vi "Auto_filename.vi"(1 "Filename Max length":i32=28, 2 "Prefix":string) -> (0 "Filename":string)   [LabVIEW 2020]
uses:
  Results_plotter_Global.vi
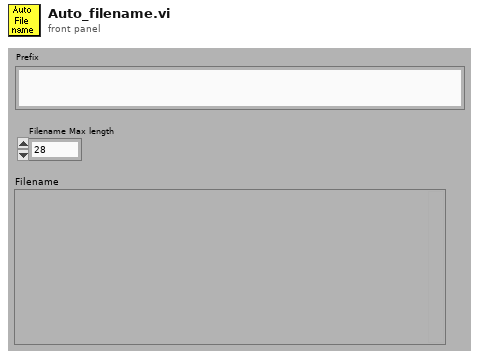
[diagram p1: front panel]
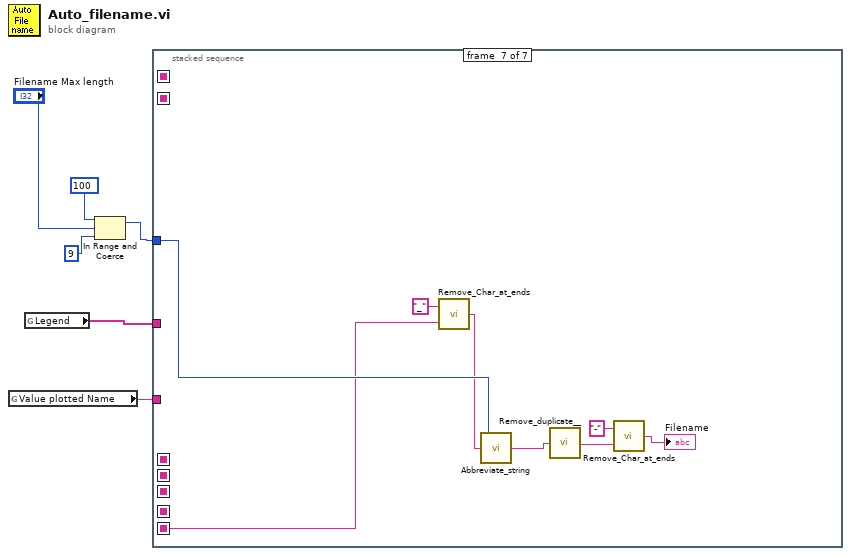
[diagram p0: block diagram]
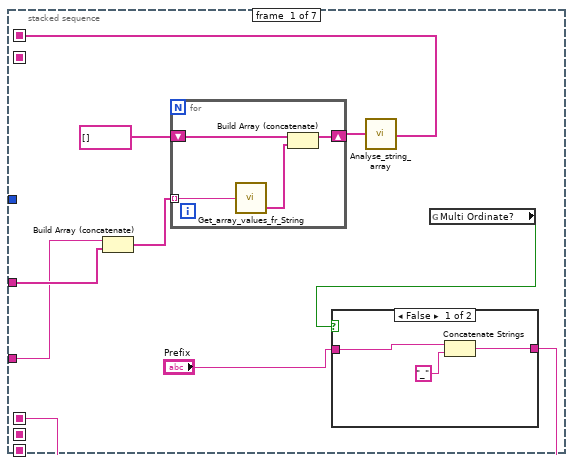
[diagram p2: hidden frame]
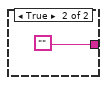
[diagram p3: hidden frame]
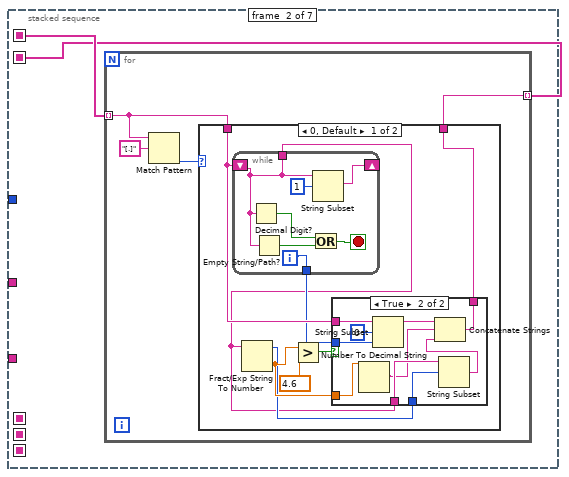
[diagram p4: hidden frame]
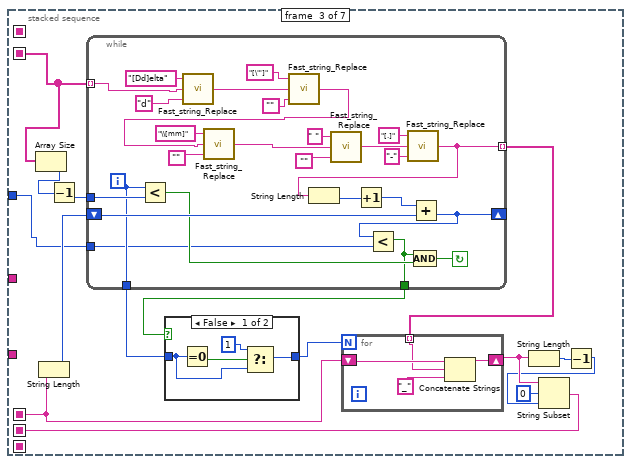
[diagram p7: hidden frame]
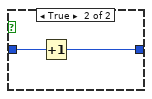
[diagram p8: hidden frame]
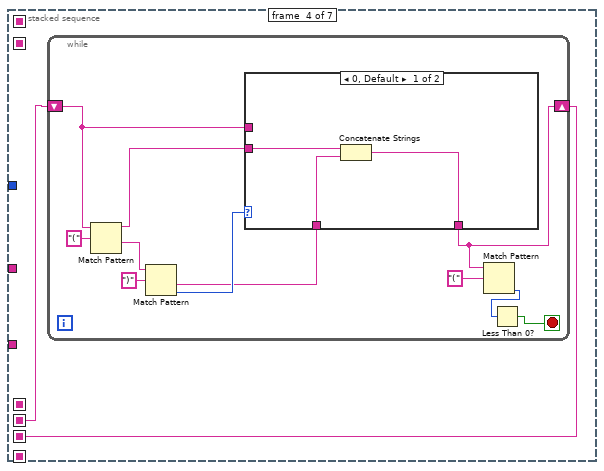
[diagram p9: hidden frame]
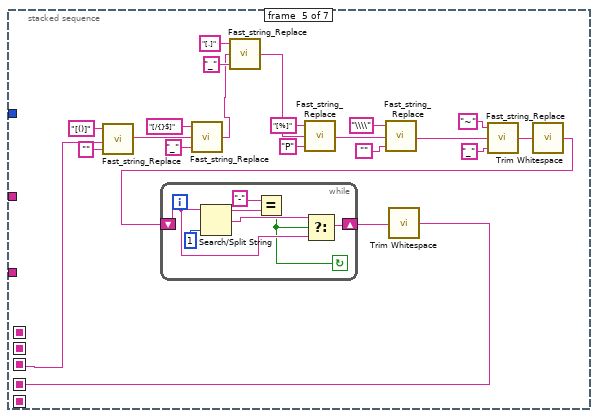
[diagram p11: hidden frame]
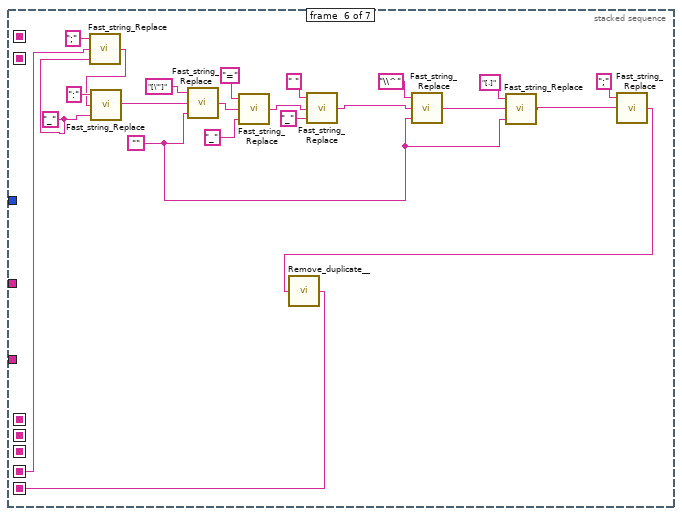
[diagram p12: hidden frame]
diagram:
  n1 = global read "Results_plotter_Global.vi" "Value plotted Name"() -> (w5:string)
  n2 = global read "Results_plotter_Global.vi" "Legend"() -> (w6:string[])
  n3 = In Range and Coerce(upper limit=100 ("length (rest)"), x="Filename Max length", lower limit=9) -> (coerced(x)=w1:i32)  [unwired: 1 out]
  n4 = stacked-sequence {
    seq-local: [_ w24 _ _ _ _ _] -> [_ _ w70 _ _ _ _]
    seq-local: [w13 _ _ _ _ _ _] -> [_ w25 _ _ _ _ _]
    seq-local: [w11 _ _ _ _ _ _] -> [_ _ w63 _ _ _ _]
    seq-local: [_ _ _ w108 _ _ _] -> [_ _ _ _ w139 _ _]
    seq-local: [_ _ _ _ w145 _ _] -> [_ _ _ _ _ w161 _]
    seq-local: [_ _ w57 _ _ _ _] -> [_ _ _ w109 _ _ _]
    seq-local: [_ _ _ _ _ w166 _] -> [_ _ _ _ _ _ w176]
    tunnel: w6 -> [w9 _ _ _ _ _ _]
    tunnel: w5 -> [w8 _ _ _ _ _ _]
    tunnel: w1 -> [_ _ w58 _ _ _ w183]
    frame #0 {
      n5 = Build Array (concatenate)(w8, w9) -> (w7:string[])
      n6 = for {
        tunnel: w7 -> [w23] mode=indexing
        shift-right: [w21] -> w14
        shift-left: string[] [] ("String array") -> [w22]
        n7 = call "Get_array_values_fr_String.vi"("String Value"=w23) -> ("String array"=w20:string[])  [unwired: 1 out]
        n8 = Build Array (concatenate)(w22, w20) -> (w21:string[])
      }
      n9 = call "Analyse_string_array.vi"("String array"=w14) -> ("Unique strings"=w13:string[])  [unwired: 2 out]
      n10 = global read "Results_plotter_Global.vi" "Multi Ordinate?"() -> (w12:bool)
      n11 = case shown="False" w12 {
        tunnel: [w17 ""] -> w11
        tunnel: "Prefix" -> [w16 _]
        frame False {
          n12 = Concatenate Strings(w16, "_" ("string")) -> (w17:string)
        }
        frame True {
        }
      }
    }
    frame #1 {
      n13 = for {
        tunnel: w25 -> [w27] mode=indexing
        tunnel: [w26] -> w24 mode=indexing
        n14 = Match Pattern(string=w27, regular expression="[.]") -> (offset past match=w28:i32)  [unwired: 4 out]
        n15 = case shown="0, Default" w28 {
          tunnel: [w31 w56] -> w26
          tunnel: w27 -> [w35 w56]
          frame 0, Default {
            n16 = while {
              shift-right: [w54] -> _
              shift-left: w35 -> [w49]
              tunnel: [w50] -> w34
              tunnel: [w49] -> w30
              i -> [w50]
              stop <- w53 stop-if-true
              n17 = Decimal Digit?(1:w49) -> (0:w52:bool)
              n18 = Empty String/Path?(string/path=w49) -> (empty?=w51:bool)
              n19 = Or(x=w52, y=w51) -> (x .or. y?=w53:bool)
              n20 = String Subset(string=w49, offset (0)=1) -> (substring=w54:string)  [unwired: 1 out]
            }
            n21 = Fract/Exp String To Number(string=w30) -> (offset past number=w32:i32, number=w33:dbl)  [unwired: 3 out]
            n22 = Greater?(x=w33, y=4.6) -> (0:w36:bool)
            n23 = case shown="True" w36 {
              tunnel: w35 -> [w38 w47]
              tunnel: w34 -> [_ w46]
              tunnel: w33 -> [_ w45]
              tunnel: w32 -> [_ w44]
              tunnel: w30 -> [_ w43]
              tunnel: [w38 w39] -> w31
              frame False {
              }
              frame True {
                n24 = Number To Decimal String(number=w45) -> (decimal integer string=w41:string)  [unwired: 1 out]
                n25 = String Subset(string=w47, offset (0)=0, length (rest)=w46) -> (substring=w42:string)
                n26 = String Subset(string=w43, offset (0)=w44) -> (substring=w40:string)  [unwired: 1 out]
                n27 = Concatenate Strings(w42, w41, w40) -> (w39:string)
              }
            }
          }
          frame -1 {
          }
        }
      }
    }
    frame #2 {
      n28 = Array Size(array=w70) -> (size(s)=w69:i32)
      n29 = String Length(string=w63) -> (length=w71:i32)
      n30 = Decrement(x=w69) -> (x-1=w68:i32)
      n31 = while {
        tunnel: w70 -> [w88] mode=indexing
        shift-right: [w96] -> _
        shift-left: w71 -> [w98]
        tunnel: w68 -> [w97]
        tunnel: [w92] -> w67
        tunnel: [w91] -> w66
        tunnel: [w90] -> w64 mode=indexing
        tunnel: w58 -> [w82]
        i -> [w91]
        stop <- w94 continue-if-true
        n32 = Less?(x=w91, y=w97) -> (x < y?=w93:bool)
        n33 = call "Fast_string_Replace.vi"("Replace match with:"="d", "Input String"=w88, "regular expression"="[Dd]elta") -> ("Output String"=w85:string)  [unwired: 2 out]
        n34 = call "Fast_string_Replace.vi"("Replace match with:"="", "Input String"=w85, "regular expression"="[\"']") -> ("Output String"=w83:string)  [unwired: 2 out]
        n35 = call "Fast_string_Replace.vi"("Replace match with:"="", "Input String"=w83, "regular expression"="\\[mm]") -> ("Output String"=w103:string)  [unwired: 2 out]
        n36 = call "Fast_string_Replace.vi"("Replace match with:"="", "Input String"=w103, "regular expression"=" ") -> ("Output String"=w101:string)  [unwired: 2 out]
        n37 = call "Fast_string_Replace.vi"("Replace match with:"="-", "Input String"=w101, "regular expression"="[.]") -> ("Output String"=w90:string)  [unwired: 2 out]
        n38 = String Length(string=w90) -> (length=w99:i32)
        n39 = Increment(x=w99) -> (x+1=w95:i32)
        n40 = Add(x=w95, y=w98) -> (x+y=w96:i32)
        n41 = Less?(x=w96, y=w82) -> (x < y?=w92:bool)
        n42 = Compound Arithmetic op=AND(w92, w93) -> (w94:bool)
      }
      n43 = case shown="False" w67 {
        tunnel: [w76 w80] -> w65
        tunnel: w66 -> [w78 w81]
        frame False {
          n44 = Equal To 0?(x=w78) -> (x = 0?=w79:bool)
          n45 = Select(t=1, s=w79, f=w78) -> (s? t:f=w76:i32)
        }
        frame True {
          n46 = Increment(x=w81) -> (x+1=w80:i32)
        }
      }
      n47 = for {
        N: w65 -> [_]
        shift-right: [w72] -> w61
        shift-left: w63 -> [w75]
        tunnel: w64 -> [w74] mode=indexing
        n48 = Concatenate Strings(w75, w74, "_" ("string")) -> (w72:string)
      }
      n49 = String Length(string=w61) -> (length=w62:i32)
      n50 = Decrement(x=w62) -> (x-1=w59:i32)
      n51 = String Subset(string=w61, offset (0)=0, length (rest)=w59) -> (substring=w57:string)
    }
    frame #3 {
      n52 = while {
        shift-right: [w112] -> w108
        shift-left: w109 -> [w114]
        stop <- w110 stop-if-true
        n53 = Match Pattern(string=w114, regular expression="(") -> (before substring=w116:string, after substring=w118:string)  [unwired: 3 out]
        n54 = Match Pattern(string=w118, regular expression=")") -> (after substring=w115:string, offset past match=w117:i32)  [unwired: 3 out]
        n55 = case shown="0, Default" w117 {
          tunnel: [w121 w124] -> w112
          tunnel: w114 -> [_ w124]
          tunnel: w116 -> [w123 _]
          tunnel: w115 -> [w122 _]
          frame 0, Default {
            n56 = Concatenate Strings(w123, w122) -> (w121:string)
          }
          frame -1 {
          }
        }
        n57 = Match Pattern(string=w112, regular expression="(") -> (offset past match=w111:i32)  [unwired: 4 out]
        n58 = Less Than 0?(x=w111) -> (x < 0?=w110:bool)
      }
    }
    frame #4 {
      n59 = call "Fast_string_Replace.vi"("Replace match with:"="", "Input String"=w139, "regular expression"="[()]") -> ("Output String"=w140:string)  [unwired: 2 out]
      n60 = call "Fast_string_Replace.vi"("Replace match with:"="_", "Input String"=w140, "regular expression"="[/{}$]") -> ("Output String"=w126:string)  [unwired: 2 out]
      n61 = call "Fast_string_Replace.vi"("Replace match with:"="_", "Input String"=w126, "regular expression"="[.]") -> ("Output String"=w125:string)  [unwired: 2 out]
      n62 = call "Fast_string_Replace.vi"("Replace match with:"="P", "Input String"=w125, "regular expression"="[%]") -> ("Output String"=w134:string)  [unwired: 2 out]
      n63 = call "Fast_string_Replace.vi"("Replace match with:"="", "Input String"=w134, "regular expression"="\\\\") -> ("Output String"=w130:string)  [unwired: 2 out]
      n64 = call "Fast_string_Replace.vi"("Replace match with:"="_", "Input String"=w130, "regular expression"="~") -> ("Output String"=w129:string)  [unwired: 2 out]
      n65 = call <vilib>:"Trim Whitespace.vi"("string"=w129) -> ("trimmed string"=w138:string)  [unwired: 1 in]
      n66 = while {
        shift-left: w138 -> [w149]
        shift-right: [w147] -> w146
        stop <- w148 continue-if-true
        n67 = Search/Split String(string=w149, offset (0)=1 ("length")) -> (substring before match=w152:string, match + rest of string=w150:string)  [unwired: 2 out]
        n68 = Equal?(x="-", y=w152) -> (x = y?=w148:bool)
        n69 = Select(t=w150, s=w148, f=w149) -> (s? t:f=w147:string)
      }
      n70 = call <vilib>:"Trim Whitespace.vi"("string"=w146) -> ("trimmed string"=w145:string)  [unwired: 1 in]
    }
    frame #5 {
      w162 = "_" ("Replace match with:")
      w157 = ""
      n71 = call "Fast_string_Replace.vi"("Replace match with:"=w162, "Input String"=w161, "regular expression"=";") -> ("Output String"=w160:string)  [unwired: 2 out]
      n72 = call "Fast_string_Replace.vi"("Replace match with:"=w162, "Input String"=w160, "regular expression"=":") -> ("Output String"=w171:string)  [unwired: 2 out]
      n73 = call "Fast_string_Replace.vi"("Replace match with:"=w157, "Input String"=w171, "regular expression"="[\"']") -> ("Output String"=w168:string)  [unwired: 2 out]
      n74 = call "Fast_string_Replace.vi"("Replace match with:"="_", "Input String"=w168, "regular expression"="=") -> ("Output String"=w167:string)  [unwired: 2 out]
      n75 = call "Fast_string_Replace.vi"("Replace match with:"="_", "Input String"=w167, "regular expression"=" ") -> ("Output String"=w164:string)  [unwired: 2 out]
      n76 = call "Fast_string_Replace.vi"("Replace match with:"=w157, "Input String"=w164, "regular expression"="\\^") -> ("Output String"=w158:string)  [unwired: 2 out]
      n77 = call "Fast_string_Replace.vi"("Replace match with:"=w157, "Input String"=w158, "regular expression"="[.]") -> ("Output String"=w155:string)  [unwired: 2 out]
      n78 = call "Fast_string_Replace.vi"("Input String"=w155, "regular expression"=";") -> ("Output String"=w154:string)  [unwired: 1 in, 2 out]
      n79 = call "Remove_duplicate__.vi"("Output String"=w154) -> ("String"=w166:string)
    }
    frame #6 {
      n80 = call "Remove_Char_at_ends.vi"("String in"=w176, "Characters to remove"="_" ("Character to remove")) -> ("String out"=w182:string)
      n81 = call "Abbreviate_string.vi"("Input String"=w182, "Max String Length"=w183) -> ("Output String"=w181:string)  [unwired: 1 in, 2 out]
      n82 = call "Remove_duplicate__.vi"("Output String"=w181) -> ("String"=w178:string)
      n83 = call "Remove_Char_at_ends.vi"("String in"=w178, "Characters to remove"="-" ("Character to remove")) -> ("String out"=→"Filename":string)
    }
  }
